vi "AlGaInPAs_v01_error.vi"(2 "Debug Mode":bool, 3 "Elapsed Time (s)":dbl, 4 "State":enum16{"Edit", "Start", "Run", "End", "Idle"}(ring), 5 "Argument List In":string[](array[string])) -> (0 "Status Out":string, 1 "Argument List Out":string[](array[string]))   [LabVIEW 2011]
panel:
  in  "Tab Control":enum32{"Al", "Ga", "In", "P", "As"}(tab)
  in  "Al Run":bool
  in  "Flow (0-100 sscm)":dbl format="%.1f"
  in  "Dilution factor":dbl min=0.0 max=10.0 format="%.2f"
  in  "Ga Run":bool
  in  "Flow (0-10 sscm)":dbl format="%.2f"
  in  "Flow (0-100 sscm)":dbl format="%.1f"
  in  "In run":bool
  in  "Flow (0-100 sccm)":dbl format="%.1f"
  in  "PH3 Run":bool
  in  "AsH3 Run":bool
  in  "Flow (0-10 sccm)":dbl format="%.2f"
  out "Al?":bool
  out "In?":bool
  out "Ga?":bool
  out "AsH3?":bool
  out "PH3?":bool
  in  "Cancel":bool
  in  "OK":bool
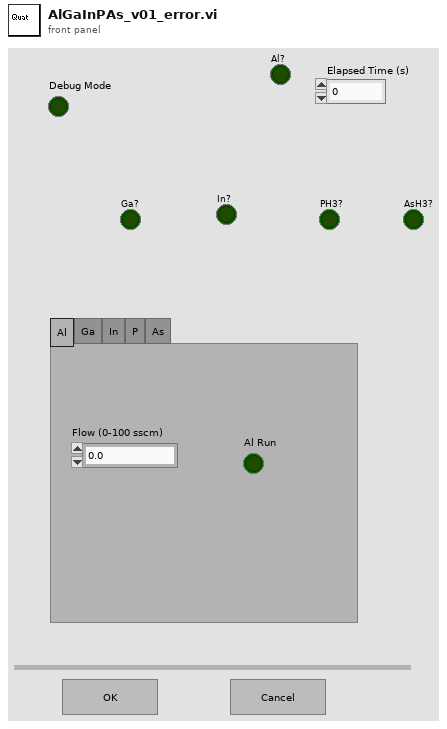
[diagram p1: front panel]
types:
  T1 = enum16{"Discrete", "Continuous", "Instantaneous"}
  T2 = enum32{"Invalid", "Default", "Floating", "Floating/Auto-Hide", "Modal"}
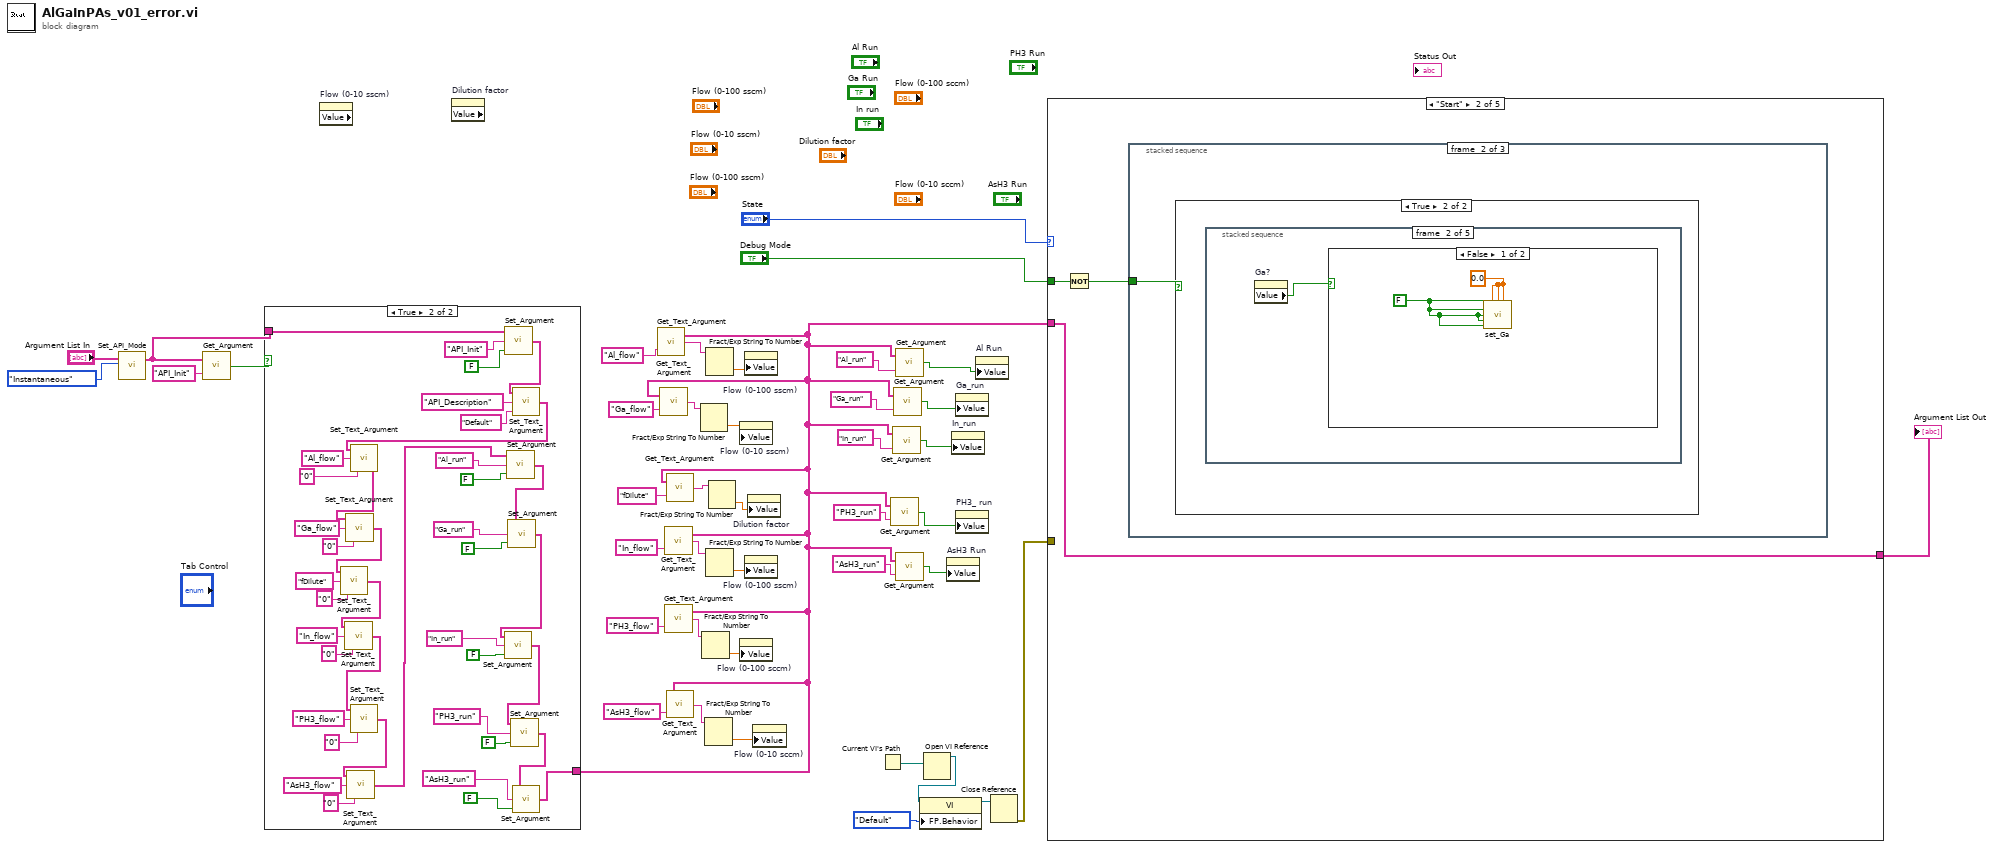
[diagram p0: block diagram]
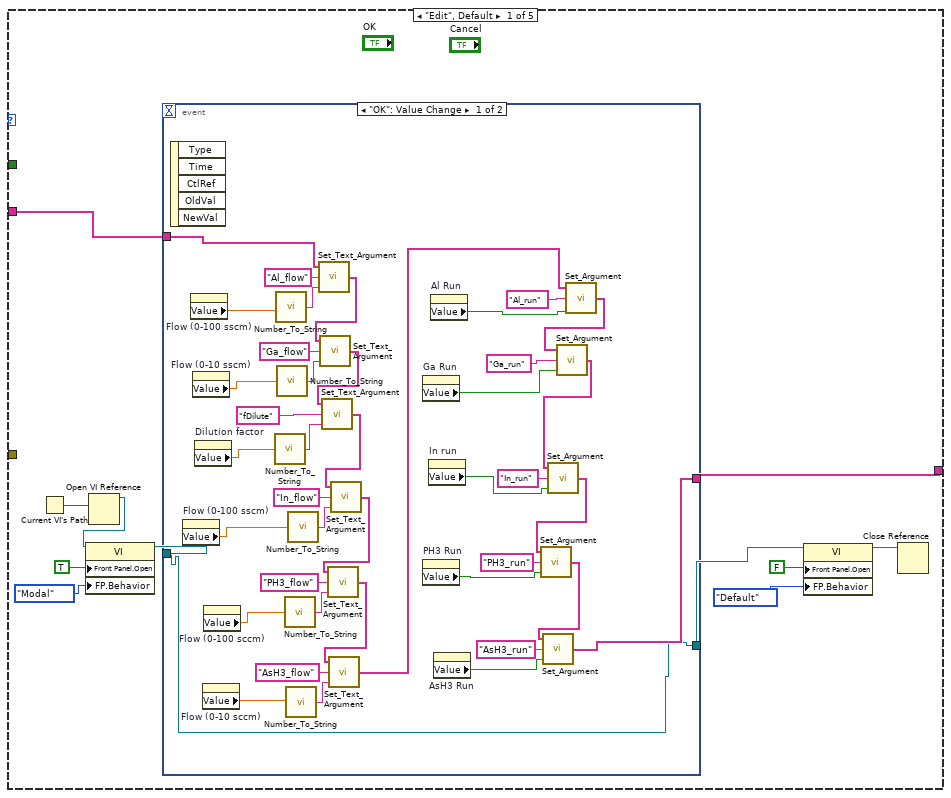
[diagram p3: hidden frame]
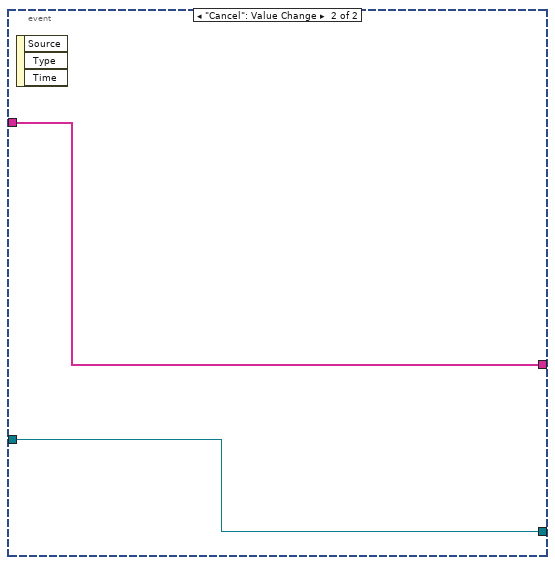
[diagram p4: hidden frame]
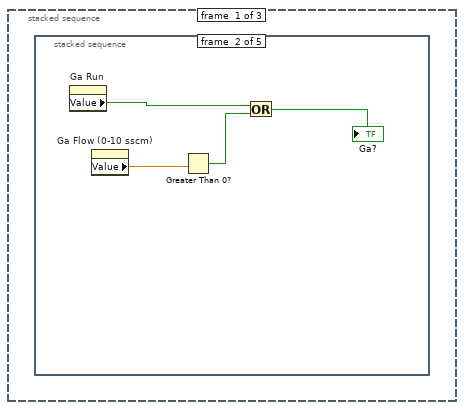
[diagram p5: hidden frame]
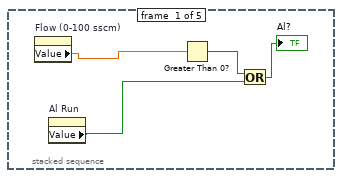
[diagram p6: hidden frame]
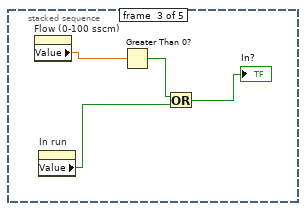
[diagram p7: hidden frame]
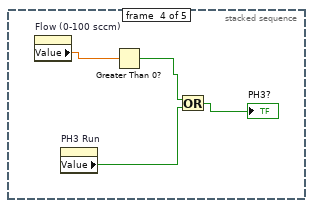
[diagram p8: hidden frame]
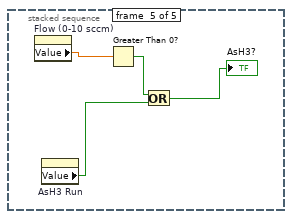
[diagram p9: hidden frame]
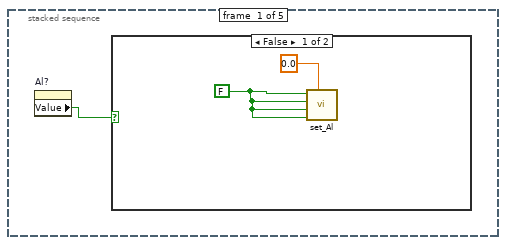
[diagram p11: hidden frame]
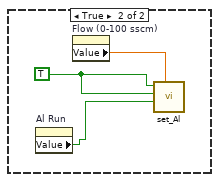
[diagram p12: hidden frame]
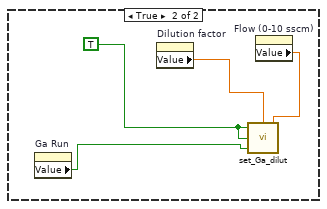
[diagram p13: hidden frame]
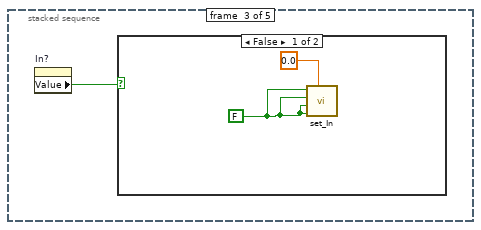
[diagram p14: hidden frame]
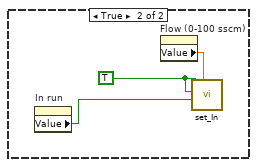
[diagram p15: hidden frame]
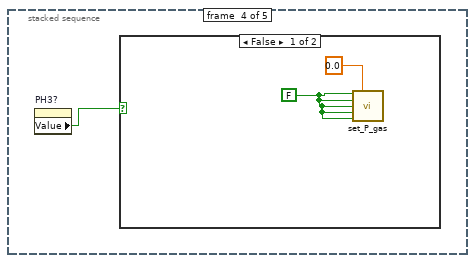
[diagram p16: hidden frame]
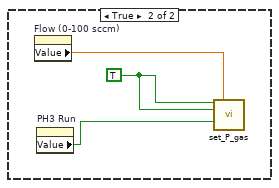
[diagram p17: hidden frame]
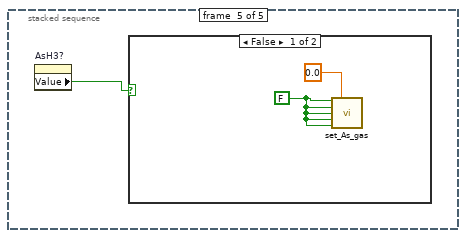
[diagram p18: hidden frame]
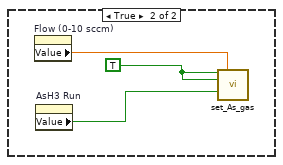
[diagram p19: hidden frame]
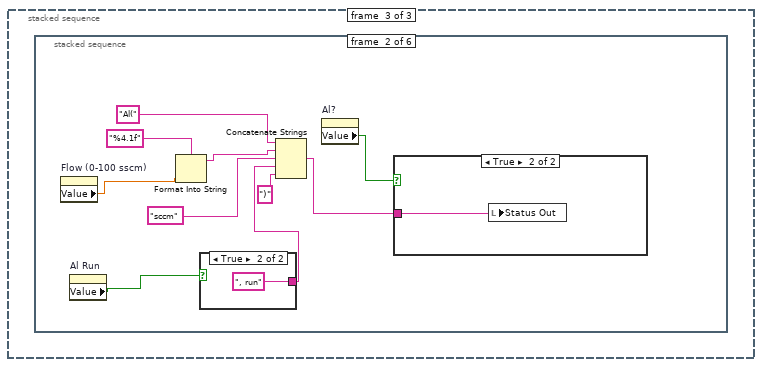
[diagram p20: hidden frame]
diagram:
  n1 = call "Set_API_Mode.vi"("API Mode"=T1."Instantaneous", "Argument List In"="Argument List In") -> ("Argument List Out"=w29:string[])  [unwired: 3 in]
  n2 = call "Get_Argument.vi"("Argument"="API_Init", "Argument List"=w29) -> ("Enabled"=w30:bool)
  n3 = case shown="True" w30 {
    tunnel: w29 -> [w43 w83]
    tunnel: [w43 w60] -> w1
    frame False {
    }
    frame True {
      n4 = call "Set_Argument.vi"("Enable"=FALSE, "Argument"="API_Init", "Argument List In"=w83) -> ("Argument List Out"=w80:string[])
      n5 = call "Set_Text_Argument.vi"("Text"="Default", "Argument"="API_Description", "Argument List In"=w80) -> ("Argument List Out"=w52:string[])
      n6 = call "Set_Text_Argument.vi"("Text"="0", "Argument"="Al_flow", "Argument List In"=w52) -> ("Argument List Out"=w51:string[])
      n7 = call "Set_Text_Argument.vi"("Text"="0", "Argument"="Ga_flow", "Argument List In"=w51) -> ("Argument List Out"=w45:string[])
      n8 = call "Set_Text_Argument.vi"("Text"="0", "Argument"="fDilute", "Argument List In"=w45) -> ("Argument List Out"=w44:string[])
      n9 = call "Set_Text_Argument.vi"("Text"="0", "Argument"="In_flow", "Argument List In"=w44) -> ("Argument List Out"=w50:string[])
      n10 = call "Set_Text_Argument.vi"("Text"="0", "Argument"="PH3_flow", "Argument List In"=w50) -> ("Argument List Out"=w62:string[])
      n11 = call "Set_Text_Argument.vi"("Text"="0", "Argument"="AsH3_flow", "Argument List In"=w62) -> ("Argument List Out"=w49:string[])
      n12 = call "Set_Argument.vi"("Enable"=FALSE, "Argument"="Al_run", "Argument List In"=w49) -> ("Argument List Out"=w55:string[])
      n13 = call "Set_Argument.vi"("Enable"=FALSE, "Argument"="Ga_run", "Argument List In"=w55) -> ("Argument List Out"=w65:string[])
      n14 = call "Set_Argument.vi"("Enable"=FALSE, "Argument"="In_run", "Argument List In"=w65) -> ("Argument List Out"=w48:string[])
      n15 = call "Set_Argument.vi"("Enable"=FALSE, "Argument"="PH3_run", "Argument List In"=w48) -> ("Argument List Out"=w58:string[])
      n16 = call "Set_Argument.vi"("Enable"=FALSE, "Argument"="AsH3_run", "Argument List In"=w58) -> ("Argument List Out"=w60:string[])
    }
  }
  n17 = property on="Flow (0-10 sscm)" class="DigNum (strict)" props=["Value"]() -> ()  [unwired: 2 in, 3 out]
  n18 = property on="Dilution factor" class="DigNum (strict)" props=["Value"]() -> ()  [unwired: 2 in, 3 out]
  n19 = call "Get_Text_Argument.vi"("Argument"="Al_flow", "Argument List"=w1) -> ("Text"=w9:string)
  n20 = call "Get_Text_Argument.vi"("Argument"="Ga_flow", "Argument List"=w1) -> ("Text"=w25:string)
  n21 = call "Get_Text_Argument.vi"("Argument"="In_flow", "Argument List"=w1) -> ("Text"=w23:string)
  n22 = call "Get_Text_Argument.vi"("Argument"="PH3_flow", "Argument List"=w1) -> ("Text"=w20:string)
  n23 = call "Get_Text_Argument.vi"("Argument"="fDilute", "Argument List"=w1) -> ("Text"=w3:string)
  n24 = call "Get_Text_Argument.vi"("Argument"="AsH3_flow", "Argument List"=w1) -> ("Text"=w21:string)
  n25 = Fract/Exp String To Number(string=w25) -> (number=w24:dbl)  [unwired: 4 out]
  n26 = Fract/Exp String To Number(string=w20) -> (number=w19:dbl)  [unwired: 4 out]
  n27 = Fract/Exp String To Number(string=w21) -> (number=w7:dbl)  [unwired: 4 out]
  n28 = Fract/Exp String To Number(string=w9) -> (number=w6:dbl)  [unwired: 4 out]
  n29 = Fract/Exp String To Number(string=w23) -> (number=w22:dbl)  [unwired: 4 out]
  n30 = Fract/Exp String To Number(string=w3) -> (number=w2:dbl)  [unwired: 4 out]
  n31 = property on="Flow (0-10 sscm)" class="DigNum (strict)"("Value"=w24) -> ()  [unwired: 2 in, 2 out]
  n32 = property on="Flow (0-100 sccm)" class="DigNum (strict)"("Value"=w19) -> ()  [unwired: 2 in, 2 out]
  n33 = property on="Flow (0-100 sscm)" class="DigNum (strict)"("Value"=w6) -> ()  [unwired: 2 in, 2 out]
  n34 = property on="Flow (0-100 sscm)" class="DigNum (strict)"("Value"=w22) -> ()  [unwired: 2 in, 2 out]
  n35 = property on="Dilution factor" class="DigNum (strict)"("Value"=w2) -> ()  [unwired: 2 in, 2 out]
  n36 = property on="Flow (0-10 sccm)" class="DigNum (strict)"("Value"=w7) -> ()  [unwired: 2 in, 2 out]
  n37 = Current VI's Path() -> (path=w38:path)
  n38 = call "Get_Argument.vi"("Argument"="PH3_run", "Argument List"=w1) -> ("Enabled"=w15:bool)
  n39 = call "Get_Argument.vi"("Argument"="In_run", "Argument List"=w1) -> ("Enabled"=w16:bool)
  n40 = call "Get_Argument.vi"("Argument"="Ga_run", "Argument List"=w1) -> ("Enabled"=w17:bool)
  n41 = call "Get_Argument.vi"("Argument"="Al_run", "Argument List"=w1) -> ("Enabled"=w5:bool)
  n42 = call "Get_Argument.vi"("Argument"="AsH3_run", "Argument List"=w1) -> ("Enabled"=w8:bool)
  n43 = Open VI Reference(vi path=w38) -> (vi reference=w37:refnum<vi>)  [unwired: 1 in, 5 out]
  n44 = property class="VI"(reference=w37, "FP.Behavior"=T2."Default" ("Front Panel Window:Behavior")) -> (reference out=w35:refnum<vi>)  [unwired: 1 in, 1 out]
  n45 = property on="AsH3 Run" class="Bool (strict)"("Value"=w8) -> ()  [unwired: 2 in, 2 out]
  n46 = property on="In_run" class="Bool (strict)"("Value"=w16) -> ()  [unwired: 2 in, 2 out]
  n47 = property on="Ga_run" class="Bool (strict)"("Value"=w17) -> ()  [unwired: 2 in, 2 out]
  n48 = property on="PH3_ run" class="Bool (strict)"("Value"=w15) -> ()  [unwired: 2 in, 2 out]
  n49 = property on="Al Run" class="Bool (strict)"("Value"=w5) -> ()  [unwired: 2 in, 2 out]
  n50 = Close Reference(reference=w35) -> (error out=w34:errorcluster)  [unwired: 1 in]
  n51 = case shown="\"Start\"" "State" {
    tunnel: [w94 w140 w263 w264 w265] -> w41
    tunnel: w1 -> [w93 w140 w263 w264 w265]
    tunnel: "Debug Mode" -> [_ w139 _ _ _]
    tunnel: w34 -> [_ _ _ _ _]
    frame "Edit", Default {
      n52 = Current VI's Path() -> (path=w88:path)
      n53 = Open VI Reference(vi path=w88) -> (vi reference=w87:refnum<vi>)  [unwired: 1 in, 5 out]
      n54 = property class="VI"(reference=w87, "Front Panel.Open"=TRUE ("Front Panel Window:Open"), "FP.Behavior"=T2."Modal" ("Front Panel Window:Behavior")) -> (reference out=w91:refnum<vi>)  [unwired: 1 in, 1 out]
      n55 = event shown="[0] \"OK\": Value Change" {
        selector: _ -> [_ _]
        dyn-events: _ -> [_ _]
        timeout: _ -> [_ _]
        tunnel: w93 -> [w118 w136]
        tunnel: [w123 w136] -> w94
        tunnel: [w110 w137] -> w90
        tunnel: w91 -> [w110 w137]
        event "OK": Value Change {
          n56 = event-data() -> ()  [unwired: 6 out]
          n57 = property on="Flow (0-100 sscm)" class="DigNum (strict)"() -> ("Value"=w102:dbl)  [unwired: 2 in, 2 out]
          n58 = property on="Flow (0-100 sscm)" class="DigNum (strict)"() -> ("Value"=w105:dbl)  [unwired: 2 in, 2 out]
          n59 = property on="Flow (0-10 sscm)" class="DigNum (strict)"() -> ("Value"=w104:dbl)  [unwired: 2 in, 2 out]
          n60 = property on="Dilution factor" class="DigNum (strict)"() -> ("Value"=w103:dbl)  [unwired: 2 in, 2 out]
          n61 = property on="Flow (0-10 sccm)" class="DigNum (strict)"() -> ("Value"=w100:dbl)  [unwired: 2 in, 2 out]
          n62 = property on="Flow (0-100 sccm)" class="DigNum (strict)"() -> ("Value"=w101:dbl)  [unwired: 2 in, 2 out]
          n63 = call "Number_To_String.vi"("Number"=w103) -> ("String"=w107:string)
          n64 = call "Number_To_String.vi"("Number"=w105) -> ("String"=w119:string)
          n65 = call "Number_To_String.vi"("Number"=w104) -> ("String"=w134:string)
          n66 = call "Number_To_String.vi"("Number"=w101) -> ("String"=w130:string)
          n67 = call "Number_To_String.vi"("Number"=w100) -> ("String"=w115:string)
          n68 = call "Number_To_String.vi"("Number"=w102) -> ("String"=w132:string)
          n69 = call "Set_Text_Argument.vi"("Text"=w119, "Argument"="Al_flow", "Argument List In"=w118) -> ("Argument List Out"=w117:string[])
          n70 = call "Set_Text_Argument.vi"("Text"=w134, "Argument"="Ga_flow", "Argument List In"=w117) -> ("Argument List Out"=w108:string[])
          n71 = call "Set_Text_Argument.vi"("Text"=w107, "Argument"="fDilute", "Argument List In"=w108) -> ("Argument List Out"=w109:string[])
          n72 = call "Set_Text_Argument.vi"("Text"=w132, "Argument"="In_flow", "Argument List In"=w109) -> ("Argument List Out"=w112:string[])
          n73 = call "Set_Text_Argument.vi"("Text"=w130, "Argument"="PH3_flow", "Argument List In"=w112) -> ("Argument List Out"=w113:string[])
          n74 = call "Set_Text_Argument.vi"("Text"=w115, "Argument"="AsH3_flow", "Argument List In"=w113) -> ("Argument List Out"=w114:string[])
          n75 = property on="Ga Run" class="Bool (strict)"() -> ("Value"=w96:bool)  [unwired: 2 in, 2 out]
          n76 = property on="PH3 Run" class="Bool (strict)"() -> ("Value"=w98:bool)  [unwired: 2 in, 2 out]
          n77 = property on="In run" class="Bool (strict)"() -> ("Value"=w97:bool)  [unwired: 2 in, 2 out]
          n78 = property on="Al Run" class="Bool (strict)"() -> ("Value"=w95:bool)  [unwired: 2 in, 2 out]
          n79 = property on="AsH3 Run" class="Bool (strict)"() -> ("Value"=w99:bool)  [unwired: 2 in, 2 out]
          n80 = call "Set_Argument.vi"("Enable"=w95, "Argument"="Al_run", "Argument List In"=w114) -> ("Argument List Out"=w111:string[])
          n81 = call "Set_Argument.vi"("Enable"=w96, "Argument"="Ga_run", "Argument List In"=w111) -> ("Argument List Out"=w126:string[])
          n82 = call "Set_Argument.vi"("Enable"=w97, "Argument"="In_run", "Argument List In"=w126) -> ("Argument List Out"=w121:string[])
          n83 = call "Set_Argument.vi"("Enable"=w98, "Argument"="PH3_run", "Argument List In"=w121) -> ("Argument List Out"=w122:string[])
          n84 = call "Set_Argument.vi"("Enable"=w99, "Argument"="AsH3_run", "Argument List In"=w122) -> ("Argument List Out"=w123:string[])
        }
        event "Cancel": Value Change {
          n85 = event-data() -> ()  [unwired: 4 out]
        }
      }
      n86 = property class="VI"(reference=w90, "Front Panel.Open"=FALSE ("Front Panel Window:Open"), "FP.Behavior"=T2."Default" ("Front Panel Window:Behavior")) -> (reference out=w84:refnum<vi>)  [unwired: 1 in, 1 out]
      n87 = Close Reference(reference=w84) -> ()  [unwired: 1 in, 1 out]
    }
    frame "Start" {
      n88 = Not(x=w139) -> (.not. x?=w138:bool)
      n89 = stacked-sequence {
        tunnel: w138 -> [_ w161 _]
        frame #0 {
          n90 = stacked-sequence {
            frame #0 {
              n91 = property on="Flow (0-100 sscm)" class="DigNum (strict)"() -> ("Value"=w142:dbl)  [unwired: 2 in, 2 out]
              n92 = property on="Al Run" class="Bool (strict)"() -> ("Value"=w141:bool)  [unwired: 2 in, 2 out]
              n93 = Greater Than 0?(x=w142) -> (x > 0?=w144:bool)
              n94 = Or(x=w144, y=w141) -> (x .or. y?=→"Al?":bool)
            }
            frame #1 {
              n95 = property on="Ga Run" class="Bool (strict)"() -> ("Value"=w147:bool)  [unwired: 2 in, 2 out]
              n96 = property on="Ga Flow (0-10 sscm)" class="DigNum (strict)"() -> ("Value"=w145:dbl)  [unwired: 2 in, 2 out]
              n97 = Greater Than 0?(x=w145) -> (x > 0?=w146:bool)
              n98 = Or(x=w147, y=w146) -> (x .or. y?=→"Ga?":bool)
            }
            frame #2 {
              n99 = property on="Flow (0-100 sscm)" class="DigNum (strict)"() -> ("Value"=w152:dbl)  [unwired: 2 in, 2 out]
              n100 = property on="In run" class="Bool (strict)"() -> ("Value"=w150:bool)  [unwired: 2 in, 2 out]
              n101 = Greater Than 0?(x=w152) -> (x > 0?=w151:bool)
              n102 = Or(x=w151, y=w150) -> (x .or. y?=→"In?":bool)
            }
            frame #3 {
              n103 = property on="Flow (0-100 sccm)" class="DigNum (strict)"() -> ("Value"=w156:dbl)  [unwired: 2 in, 2 out]
              n104 = property on="PH3 Run" class="Bool (strict)"() -> ("Value"=w154:bool)  [unwired: 2 in, 2 out]
              n105 = Greater Than 0?(x=w156) -> (x > 0?=w155:bool)
              n106 = Or(x=w155, y=w154) -> (x .or. y?=→"PH3?":bool)
            }
            frame #4 {
              n107 = property on="Flow (0-10 sccm)" class="DigNum (strict)"() -> ("Value"=w160:dbl)  [unwired: 2 in, 2 out]
              n108 = property on="AsH3 Run" class="Bool (strict)"() -> ("Value"=w158:bool)  [unwired: 2 in, 2 out]
              n109 = Greater Than 0?(x=w160) -> (x > 0?=w159:bool)
              n110 = Or(x=w159, y=w158) -> (x .or. y?=→"AsH3?":bool)
            }
          }
        }
        frame #1 {
          n111 = case shown="True" w161 {
            frame False {
            }
            frame True {
              n112 = stacked-sequence {
                frame #0 {
                  n113 = property on="Al?" class="Bool (strict)"() -> ("Value"=w162:bool)  [unwired: 2 in, 2 out]
                  n114 = case shown="False" w162 {
                    frame False {
                      w163 = FALSE ("Al Active")
                      n115 = call "set_Al.vi"("Aluminum Flow"=0.0, "Al Remote"=w163, "Al Run"=w163, "Al Bubbler"=w163, "Al Active"=w163) -> ()  [unwired: 5 out]
                    }
                    frame True {
                      w167 = TRUE ("Al Active")
                      n116 = property on="Al Run" class="Bool (strict)"() -> ("Value"=w165:bool)  [unwired: 2 in, 2 out]
                      n117 = property on="Flow (0-100 sscm)" class="DigNum (strict)"() -> ("Value"=w166:dbl)  [unwired: 2 in, 2 out]
                      n118 = call "set_Al.vi"("Aluminum Flow"=w166, "Al Run"=w165, "Al Bubbler"=w167, "Al Active"=w167) -> ()  [unwired: 1 in, 5 out]
                    }
                  }
                }
                frame #1 {
                  n119 = property on="Ga?" class="Bool (strict)"() -> ("Value"=w168:bool)  [unwired: 2 in, 2 out]
                  n120 = case shown="False" w168 {
                    frame False {
                      w170 = FALSE ("Ga Active")
                      w169 = 0.0 ("Ga Flow 1")
                      n121 = call "set_Ga.vi"("Ga Active"=w170, "Ga Flow 3"=w169, "Ga Flow 2"=w169, "Ga Flow 1"=w169, "Ga Bubbler"=w170, "Ga H2 Dilute"=w170, "Ga Run"=w170, "Ga Remote"=w170) -> ()  [unwired: 8 out]
                    }
                    frame True {
                      w173 = TRUE ("Ga Active")
                      n122 = property on="Ga Run" class="Bool (strict)"() -> ("Value"=w174:bool)  [unwired: 2 in, 2 out]
                      n123 = property on="Dilution factor" class="DigNum (strict)"() -> ("Value"=w172:dbl)  [unwired: 2 in, 2 out]
                      n124 = property on="Flow (0-10 sscm)" class="DigNum (strict)"() -> ("Value"=w171:dbl)  [unwired: 2 in, 2 out]
                      n125 = call "set_Ga_dilut.vi"("Ga flow (0-10 sccm)"=w171, "fDilution"=w172, "Run"=w174, "Bubbler In"=w173, "Active"=w173) -> ()
                    }
                  }
                }
                frame #2 {
                  n126 = property on="In?" class="Bool (strict)"() -> ("Value"=w175:bool)  [unwired: 2 in, 2 out]
                  n127 = case shown="False" w175 {
                    frame False {
                      w177 = FALSE ("In Remote")
                      n128 = call "set_In.vi"("Indium Flow"=0.0, "In Remote"=w177, "In Run"=w177, "In Bubbler"=w177, "In Active"=w177) -> ()  [unwired: 5 out]
                    }
                    frame True {
                      w180 = TRUE ("In Run")
                      n129 = property on="In run" class="Bool (strict)"() -> ("Value"=w178:bool)  [unwired: 2 in, 2 out]
                      n130 = property on="Flow (0-100 sscm)" class="DigNum (strict)"() -> ("Value"=w179:dbl)  [unwired: 2 in, 2 out]
                      n131 = call "set_In.vi"("Indium Flow"=w179, "In Run"=w178, "In Bubbler"=w180, "In Active"=w180) -> ()  [unwired: 1 in, 5 out]
                    }
                  }
                }
                frame #3 {
                  n132 = property on="PH3?" class="Bool (strict)"() -> ("Value"=w181:bool)  [unwired: 2 in, 2 out]
                  n133 = case shown="False" w181 {
                    frame False {
                      w182 = FALSE ("P_Gas Active")
                      n134 = call "set_P_gas.vi"("P_Gas Active"=w182, "P_Gas Flow"=0.0, "P_Gas In"=w182, "P_Gas H2 In"=w182, "P_Gas Run"=w182, "P_Gas Remote"=w182) -> ()  [unwired: 10 out]
                    }
                    frame True {
                      w186 = TRUE ("P_Gas Active")
                      n135 = property on="Flow (0-100 sccm)" class="DigNum (strict)"() -> ("Value"=w185:dbl)  [unwired: 2 in, 2 out]
                      n136 = property on="PH3 Run" class="Bool (strict)"() -> ("Value"=w184:bool)  [unwired: 2 in, 2 out]
                      n137 = call "set_P_gas.vi"("P_Gas Active"=w186, "P_Gas Flow"=w185, "P_Gas In"=w186, "P_Gas Run"=w184) -> ()  [unwired: 2 in, 10 out]
                    }
                  }
                }
                frame #4 {
                  n138 = property on="AsH3?" class="Bool (strict)"() -> ("Value"=w187:bool)  [unwired: 2 in, 2 out]
                  n139 = case shown="False" w187 {
                    frame False {
                      w188 = FALSE ("As_Gas Active")
                      n140 = call "set_As_gas.vi"("As_Gas Active"=w188, "As_Gas Flow"=0.0, "As_Gas In"=w188, "As_Gas H2"=w188, "As_Gas Run"=w188, "As_Gas Remote"=w188) -> ()  [unwired: 10 out]
                    }
                    frame True {
                      w192 = TRUE ("As_Gas Active")
                      n141 = property on="Flow (0-10 sccm)" class="DigNum (strict)"() -> ("Value"=w190:dbl)  [unwired: 2 in, 2 out]
                      n142 = property on="AsH3 Run" class="Bool (strict)"() -> ("Value"=w191:bool)  [unwired: 2 in, 2 out]
                      n143 = call "set_As_gas.vi"("As_Gas Active"=w192, "As_Gas Flow"=w190, "As_Gas In"=w192, "As_Gas Run"=w191) -> ()  [unwired: 2 in, 10 out]
                    }
                  }
                }
              }
            }
          }
        }
        frame #2 {
          n144 = stacked-sequence {
            frame #0 {
              n145 = local write "Status Out"("" ("Status Out")) -> ()
            }
            frame #1 {
              n146 = property on="Flow (0-100 sscm)" class="DigNum (strict)"() -> ("Value"=w195:dbl)  [unwired: 2 in, 2 out]
              n147 = property on="Al Run" class="Bool (strict)"() -> ("Value"=w194:bool)  [unwired: 2 in, 2 out]
              n148 = Format Into String(format string="%4.1f", w195) -> (resulting string=w198:string)  [unwired: 2 in, 1 out]
              n149 = case shown="True" w194 {
                tunnel: ["" ", run"] -> w201
                frame False {
                }
                frame True {
                }
              }
              n150 = Concatenate Strings("Al(" ("string"), w198, "sccm" ("string"), w201, ")" ("string")) -> (w199:string)
              n151 = property on="Al?" class="Bool (strict)"() -> ("Value"=w196:bool)  [unwired: 2 in, 2 out]
              n152 = case shown="True" w196 {
                tunnel: w199 -> [_ w204]
                frame False {
                }
                frame True {
                  n153 = local write "Status Out"(w204) -> ()
                }
              }
            }
            frame #2 {
              n154 = property on="Ga Run" class="Bool (strict)"() -> ("Value"=w209:bool)  [unwired: 2 in, 2 out]
              n155 = property on="Flow (0-10 sscm)" class="DigNum (strict)"() -> ("Value"=w210:dbl)  [unwired: 2 in, 2 out]
              n156 = Format Into String(format string="%4.1f", w210) -> (resulting string=w212:string)  [unwired: 2 in, 1 out]
              n157 = case shown="True" w209 {
                tunnel: ["" ", run"] -> w215
                frame False {
                }
                frame True {
                }
              }
              n158 = property on="Status Out" class="Str"() -> ("Value"=w207:string)  [unwired: 2 in, 2 out]
              n159 = Concatenate Strings(w207, "Ga(" ("string"), w212, "sccm" ("string"), w215, ")" ("string")) -> (w213:string)
              n160 = property on="Ga?" class="Bool (strict)"() -> ("Value"=w208:bool)  [unwired: 2 in, 2 out]
              n161 = case shown="True" w208 {
                tunnel: w213 -> [_ w218]
                frame False {
                }
                frame True {
                  n162 = local write "Status Out"(w218) -> ()
                }
              }
            }
            frame #3 {
              n163 = property on="In run" class="Bool (strict)"() -> ("Value"=w223:bool)  [unwired: 2 in, 2 out]
              n164 = property on="Flow (0-100 sscm)" class="DigNum (strict)"() -> ("Value"=w224:dbl)  [unwired: 2 in, 2 out]
              n165 = Format Into String(format string="%4.1f", w224) -> (resulting string=w226:string)  [unwired: 2 in, 1 out]
              n166 = property on="Status Out" class="Str"() -> ("Value"=w221:string)  [unwired: 2 in, 2 out]
              n167 = case shown="False" w223 {
                tunnel: ["" ", run"] -> w229
                frame False {
                }
                frame True {
                }
              }
              n168 = Concatenate Strings(w221, "In(" ("string"), w226, "sccm" ("string"), w229, ")" ("string")) -> (w227:string)
              n169 = property on="In?" class="Bool (strict)"() -> ("Value"=w222:bool)  [unwired: 2 in, 2 out]
              n170 = case shown="True" w222 {
                tunnel: w227 -> [_ w232]
                frame False {
                }
                frame True {
                  n171 = local write "Status Out"(w232) -> ()
                }
              }
            }
            frame #4 {
              n172 = property on="PH3 Run" class="Bool (strict)"() -> ("Value"=w238:bool)  [unwired: 2 in, 2 out]
              n173 = property on="Flow (0-100 sccm)" class="DigNum (strict)"() -> ("Value"=w239:dbl)  [unwired: 2 in, 2 out]
              n174 = Format Into String(format string="%4.1f", w239) -> (resulting string=w241:string)  [unwired: 2 in, 1 out]
              n175 = case shown="False" w238 {
                tunnel: ["" ", run"] -> w243
                frame False {
                }
                frame True {
                }
              }
              n176 = property on="Status Out" class="Str"() -> ("Value"=w236:string)  [unwired: 2 in, 2 out]
              n177 = Concatenate Strings(w236, "PH3(" ("string"), w241, "sccm" ("string"), w243, ")" ("string")) -> (w237:string)
              n178 = property on="PH3?" class="Bool (strict)"() -> ("Value"=w240:bool)  [unwired: 2 in, 2 out]
              n179 = case shown="True" w240 {
                tunnel: w237 -> [_ w246]
                frame False {
                }
                frame True {
                  n180 = local write "Status Out"(w246) -> ()
                }
              }
            }
            frame #5 {
              n181 = property on="AsH3 Run" class="Bool (strict)"() -> ("Value"=w252:bool)  [unwired: 2 in, 2 out]
              n182 = property on="Flow (0-10 sccm)" class="DigNum (strict)"() -> ("Value"=w253:dbl)  [unwired: 2 in, 2 out]
              n183 = Format Into String(format string="%4.2f", w253) -> (resulting string=w254:string)  [unwired: 2 in, 1 out]
              n184 = case shown="True" w252 {
                tunnel: ["" ", run"] -> w257
                frame False {
                }
                frame True {
                }
              }
              n185 = property on="Status Out" class="Str"() -> ("Value"=w250:string)  [unwired: 2 in, 2 out]
              n186 = Concatenate Strings(w250, "AsH3(" ("string"), w254, "sccm" ("string"), w257, ")" ("string")) -> (w255:string)
              n187 = property on="AsH3?" class="Bool (strict)"() -> ("Value"=w251:bool)  [unwired: 2 in, 2 out]
              n188 = case shown="True" w251 {
                tunnel: w255 -> [_ w260]
                frame False {
                }
                frame True {
                  n189 = local write "Status Out"(w260) -> ()
                }
              }
            }
          }
        }
      }
    }
    frame "Run" {
    }
    frame "End" {
    }
    frame "Idle" {
    }
  }
  "Argument List Out" <- w41
